vi "AVI-read frame period.vi"(8 "error in (no error)":errorcluster) -> (0 "error out":errorcluster, 2 "Frame period (ms)":dbl)   [LabVIEW 2013]
uses:
  Globals/gl_Time series viewer globals.vi
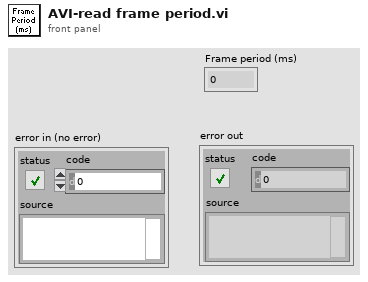
[diagram p1: front panel]
types:
  T1 = typedef "AVI playback header info cluster.ctl" = cluster{"Frame Size":u32, "AOD fill time (us)":dbl, "Dwell time (us)":dbl, "Frame period (ms)":dbl, "Number of Miniscans":u16, "Number of Pixels in Miniscan":u16}
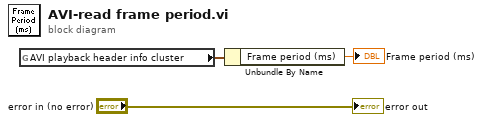
[diagram p0: block diagram]
diagram:
  n1 = global read "gl_Time series viewer globals.vi" "AVI playback header info cluster"() -> (w2:T1)
  n2 = Unbundle By Name(w2) -> ("Frame period (ms)"=→"Frame period (ms)":dbl)
  "error out" <- "error in (no error)"
